vi "Write.vi"(5 "port or service name":u16, 7 "IP":string, 8 "error in (no error)":errorcluster, 9 "timeout ms (25000)":i32=2000, 10 "data in":string, 11 "connection ID":refnum<k16>) -> (0 "error out":errorcluster, 3 "connection ID":refnum<k16>)   [LabVIEW 2018, in "Simple UDP Message.lvlib"]
uses:
  Simple UDP Message.lvlib
panel:
  # "tx rx 2buffer"
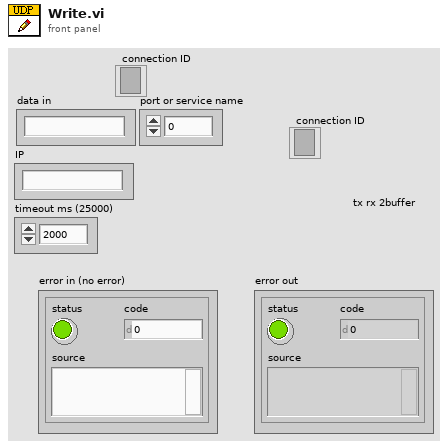
[diagram p1: front panel]
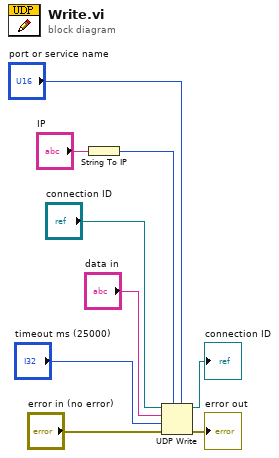
[diagram p0: block diagram]
diagram:
  n1 = String To IP(1:"IP") -> (0:w4:u32)
  n2 = UDP Write(address=w4, port or service name="port or service name", connection ID="connection ID", data in="data in", 8:"error in (no error)", 9:"timeout ms (25000)") -> (error out=→"error out":errorcluster, 3:→"connection ID":refnum<k16>)
